vi "Write_Csv_Erds (Only Name and Erds).vi"(0 "Refnum_In_Csv":refnum<file>, 5 "ERD Name Array In":string[](array[string]), 7 "ERD Number Array In":string[](array[string]), 9 "Data_Erd_Read":string[](array[string]), 11 "Write Header ? In":bool) -> ()   [LabVIEW 2023]
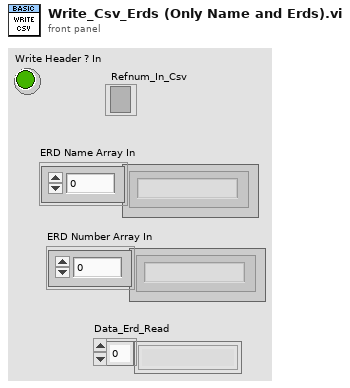
[diagram p1: front panel]
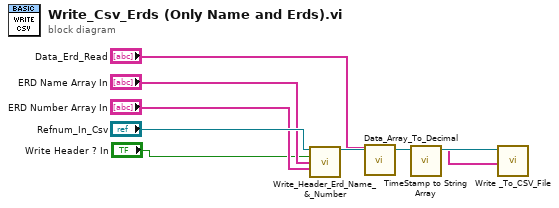
[diagram p0: block diagram]
diagram:
  n1 = call "Write_Header_Erd_Name_&_Number.vi"("Refnum_In_Csv"="Refnum_In_Csv", "Write_Header?"="Write Header ? In", "ERD Name Array In"="ERD Name Array In", "ERD Number Array In"="ERD Number Array In") -> ("Refnum_Out_Csv"=w8:refnum<file>)  [unwired: 11 in]
  n2 = call "Data_Array_To_Decimal.vi"("Data_Erd_Read"="Data_Erd_Read") -> ("Data_Decimal"=w2:string[])  [unwired: 14 in]
  n3 = call "TimeStamp to String Array.vi"("String Array In"=w2) -> ("String Array Out"=w7:string[])  [unwired: 10 in]
  n4 = call "Write _To_CSV_File.vi"("Refnum In"=w8, "ERD Data"=w7) -> ()  [unwired: 15 in, 3 out]
